vi "Helper SubVI - Generate Chirplet.vi"(10 "parameter":T1={"alpha"=-0.009133995535746432, "t0"=50.579142909047555, "omega (rad)"=2.2274811453021033, "beta"=0.0009778377050386304} {"beta" format="%.3e"; "omega (rad)" format="%.3e"; "t0" format="%.3e"; "alpha" format="%.3e"}, 11 "length":i32=1024) -> (3 "h(t)":cdb[](array[numeric]) format="%.2f")   [LabVIEW 2023]
doc: "Generates Chirplet according to Chirplet parameters."
uses:
  <vilib>/Analysis/1siggen.llb/Ramp Pattern by Samples.vi
  <vilib>/Analysis/NI_AALBase.lvlib
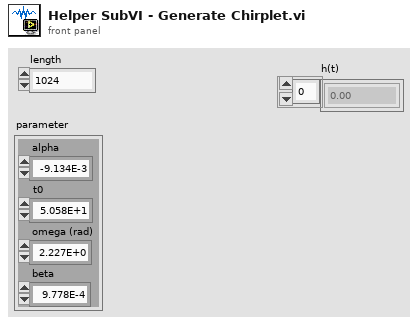
[diagram p1: front panel]
types:
  T1 = cluster{"alpha":dbl, "t0":dbl, "omega (rad)":dbl, "beta":dbl}
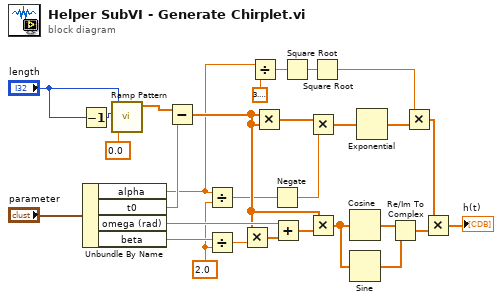
[diagram p0: block diagram]
diagram:
  w15 = 2.0 ("y")
  n1 = Decrement(x="length") -> (x-1=w28:i32)
  n2 = Unbundle By Name("parameter") -> ("alpha"=w4:dbl, "t0"=w21:dbl, "omega (rad)"=w17:dbl, "beta"=w20:dbl)
  n3 = call-poly <vilib>:"Ramp Pattern.vi"("start"=0.0, "end"=w28, "samples"="length") -> ("Ramp Pattern"=w22:dbl[])  [unwired: 7 in, 1 out]
  n4 = Subtract(x=w22, y=w21) -> (x-y=w14:dbl[])
  n5 = Divide(x=w4, y=w15) -> (x/y=w12:dbl)
  n6 = Divide(x=w20, y=w15) -> (x/y=w19:dbl)
  n7 = Multiply(x=w14, y=w19) -> (x*y=w18:dbl[])
  n8 = Divide(x=w4, y=3.141592653589793 ("Pi")) -> (x/y=w24:dbl)
  n9 = Multiply(x=w14, y=w14) -> (x*y=w13:dbl[])
  n10 = Negate(x=w12) -> (-x=w11:dbl)
  n11 = Add(x=w17, y=w18) -> (x+y=w16:dbl[])
  n12 = Square Root(x=w24) -> (sqrt(x)=w23:dbl)
  n13 = Multiply(x=w13, y=w11) -> (x*y=w10:dbl[])
  n14 = Multiply(x=w14, y=w16) -> (x*y=w9:dbl[])
  n15 = Square Root(x=w23) -> (sqrt(x)=w3:dbl)
  n16 = Cosine(x=w9) -> (cos(x)=w8:dbl[])
  n17 = Sine(x=w9) -> (sin(x)=w7:dbl[])
  n18 = Exponential(1:w10) -> (0:w5:dbl[])
  n19 = Re/Im To Complex(1:w7, 2:w8) -> (0:w6:cdb[])
  n20 = Multiply(x=w3, y=w5) -> (x*y=w2:dbl[])
  n21 = Multiply(x=w2, y=w6) -> (x*y=→"h(t)":cdb[])
